vi "Do.vi"(8 "error in (no error)":errorcluster, 10 "Actor in":refnum<class "Actor.lvclass">, 11 "Read Data Msg":refnum<class "Read Data Msg.lvclass">) -> (0 "error out":errorcluster, 2 "Actor out":refnum<class "Actor.lvclass">)   [LabVIEW 2025, in "PLC_Abstr.lvlib" / "Read Data Msg.lvclass"]
doc: "This VI delivers the message to the actor by calling the appropriate method(s) on the actor."
uses:
  Read Data Msg.lvclass
  <vilib>/ActorFramework/Actor/Actor.lvclass
  Read Data Msg.lvclass/Read Data Msg.ctl
  PLC_Abstr/PLC_Abstr.lvclass
  dd058554-592b-49b1-bae7-8f067c580f40.vi
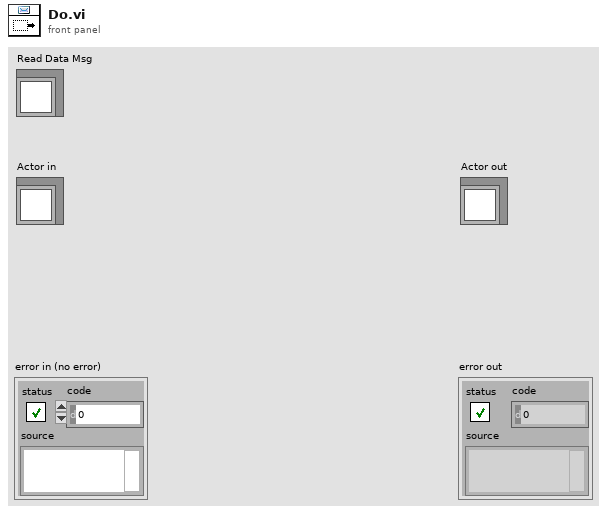
[diagram p1: front panel]
types:
  T1 = typedef "PLC_Module.lvlib/PLC_Module.lvclass/PLC_Data_Type.ctl" = enum16{"Boolean", "Single Float", "U8", "U32", "U32_Array", "String"}
  T2 = cluster{"Data":variant, "error out":errorcluster}
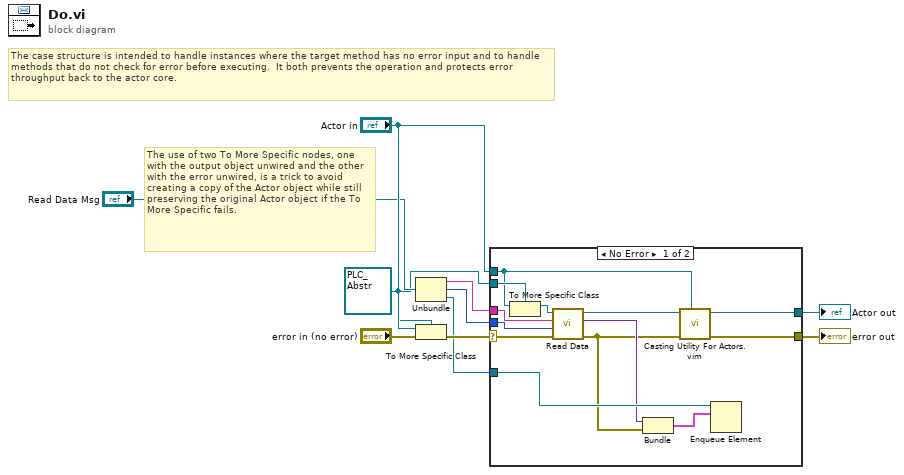
[diagram p0: block diagram]
diagram:
  w5 = refnum<class "PLC_Abstr.lvclass"> refnum ("Actor in")
  # "The use of two To More Specific nodes, one with the output object unwired and the other with the error unwired, is a trick to avoid creating a copy of the Actor object while still preserving the original Actor object if the To More Specific fails."
  # "The case structure is intended to handle instances where the target method has no error input and to handle methods that do not check for error before executing.  It both prevents the operation and protects error throughput back to the actor core."
  n1 = Unbundle("Read Data Msg") -> (w3:string, w2:T1, w1:refnum<queue>)
  n2 = To More Specific Class(target class=w5, reference="Actor in", error in="error in (no error)") -> (error out=w4:errorcluster)  [unwired: 1 out]
  n3 = case shown="No Error" w4 {
    selector: w4 -> [w23 w25]
    tunnel: [w17 w25] -> w10
    tunnel: [w18 w24] -> w9
    tunnel: "Actor in" -> [w20 w24]
    tunnel: w5 -> [w21 _]
    tunnel: w3 -> [w16 _]
    tunnel: w2 -> [w15 _]
    tunnel: w1 -> [w14 _]
    frame No Error {
      n4 = To More Specific Class(target class=w21, reference=w20) -> (specific class reference=w22:refnum<class "PLC_Abstr.lvclass">)  [unwired: 1 in, 1 out]
      n5 = call-dynamic "Read Data.vi"("error in (no error)"=w23, "DataType"=w15, "Address"=w16, "PLC_Abstr in"=w22) -> ("error out"=w12:errorcluster, "Data"=w13:variant, "PLC_Abstr out"=w19:refnum<class "PLC_Abstr.lvclass">)  [unwired: 5 in]
      n6 = Bundle("Data"=w13, "error out"=w12) -> (w11:T2)  [unwired: 1 in]
      n7 = call "Casting Utility For Actors.vim"("type"=w20, "error in (no error)"=w12, "Actor in"=w19) -> ("error out"=w17:errorcluster, "Actor out"=w18:refnum<class "Actor.lvclass">)  [unwired: 7 in]
      n8 = Enqueue Element(queue=w14, element=w11) -> ()  [unwired: 2 in, 3 out]
    }
    frame Error {
      # "If type check fails, pass the original object out again."
    }
  }
  "error out" <- w10
  "Actor out" <- w9
